vi "Draw 2D Plot.vi"(6 "Control Ref Queue":T1, 8 "error in (no error)":errorcluster, 10 "Multiplot Representation In":T2, 11 "2D Error Bar.lvclass in":refnum<class "2D Error Bar.lvclass">) -> (0 "error out":errorcluster, 2 "Multiplot Representation Out":T2, 3 "2D Error Bar.lvclass out":refnum<class "2D Error Bar.lvclass">)   [LabVIEW 2020, in "2D Error Bar.lvclass"]
uses:
  <vilib>/Math Plots/2D Math Plots/2D Error Bar/2D Error Bar/2D Error Bar.lvclass
  e:/builds/penguin/labview/branches/2020/dev/dist/vi.lib/Math Plots/2D Math Plots/2D Plot/2D Plot/2D Plot.lvclass
  <vilib>/Math Plots/2D Math Plots/2D Plot/2D Plot/Typedef/Multiplot Representation.ctl
  <vilib>/Math Plots/2D Math Plots/2D Plot/2D Plot/Typedef/Plot Representation.ctl
  <vilib>/Math Plots/2D Math Plots/2D Plot/2D Plot/Typedef/Range Cluster.ctl
  <vilib>/Math Plots/2D Math Plots/2D Plot/Action String/2DMathPlot Ctrl Act Queue.ctl
  <vilib>/Math Plots/2D Math Plots/2D Plot/Action String/2DMathPlot Ctrl Act Cluster.ctl
  <vilib>/Math Plots/2D Math Plots/2D Plot/Action String/2DMathPlot State Class.ctl
  <vilib>/Math Plots/2D Math Plots/2D Error Bar/2D Error Bar/2D Error Bar.lvclass/2D Error Bar.ctl
  <vilib>/Math Plots/2D Math Plots/2D Plot/2D Plot/2D Plot.lvclass
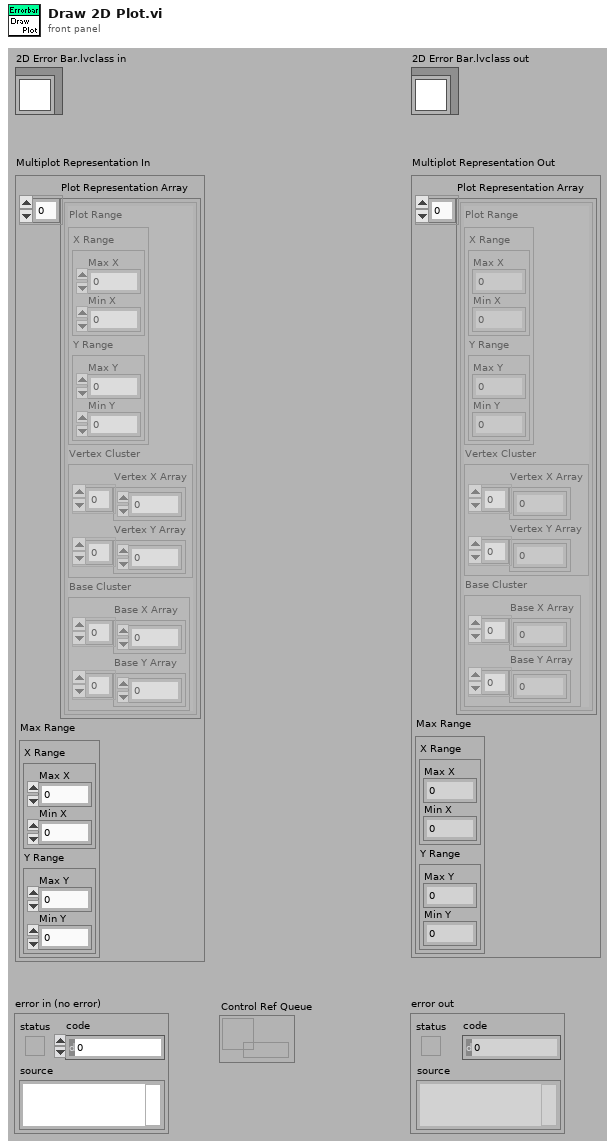
[diagram p1: front panel]
types:
  T1 = typedef "2DMathPlot Ctrl Act Queue.ctl" = refnum<queue>
  T2 = typedef "2D Plot.lvclass/Multiplot Representation.ctl" = cluster{"Plot Representation Array":T3[], "Max Range":T4}
  T3 = typedef "2D Plot.lvclass/Plot Representation.ctl" = cluster{"Plot Range":T4, "Vertex Cluster":cluster{"Vertex X Array":dbl[], "Vertex Y Array":dbl[]}, "Base Cluster":cluster{"Base X Array":dbl[], "Base Y Array":dbl[]}}
  T4 = typedef "2D Plot.lvclass/Range Cluster.ctl" = cluster{"X Range":cluster{"Max X":dbl, "Min X":dbl}, "Y Range":cluster{"Max Y":dbl, "Min Y":dbl}}
  T5 = typedef "2DMathPlot Ctrl Act Cluster.ctl" = cluster{"Plot Area Ref":refnum<vi>, "Z Axis Ref":refnum<vi>, "Legend Ref":refnum<vi>, "XControl Ref":refnum<vi>, "Facade Ref":refnum<vi>, "Display State Change Class":T6}
  T6 = typedef "2DMathPlot State Class.ctl" = enum16{"Update All (Undo)", "Update General", "Update Appearance", "Update Format", "Update Scale", "Update Marker", "Update Cursor", "None"}
  T7 = cluster{"Base X Array":dbl[], "Base Y Array":dbl[]}
  T8 = typedef "2D Plot.lvclass/Plot Property Array.ctl" = T9[]
  T9 = typedef "2D Plot.lvclass/Plot Property.ctl" = cluster{"Bar Plot Style":u8, "DigitalLineStyle":u8, "TransitionLocation":u8, "Transition Type":u8, "Fill To":i16, "Fill/Pt. Color":u32, "Label Style":u8, "Line Style":u8, "Line Width":u8, "Plot Color":u32, "Plot Interpolation":u8, "Plot Name":string, "Point Style":u8, "Visible?":bool, "XScaleIdx":u32, "YScaleIdx":u32}
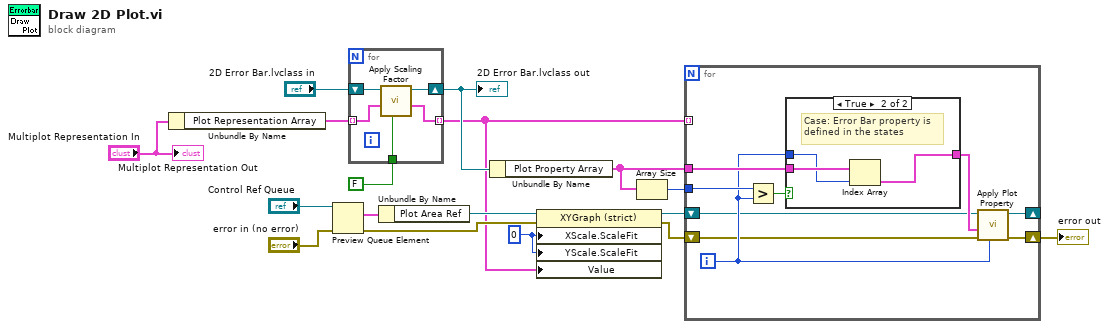
[diagram p0: block diagram]
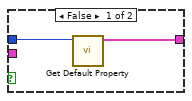
[diagram p2: hidden frame]
diagram:
  w11 = u8 0 ("X Scale.Scale Fit")
  n1 = Unbundle By Name("Multiplot Representation In") -> ("Plot Representation Array"=w5:T3[])
  n2 = Preview Queue Element(queue="Control Ref Queue", error in (no error)="error in (no error)") -> (element=w8:T5, error out=w10:errorcluster)  [unwired: 3 out]
  n3 = for {
    tunnel: w5 -> [w22] mode=indexing
    tunnel: [w18] -> w1 mode=indexing
    tunnel: FALSE ("Plot Image?") -> [w21]
    shift-right: [w19] -> w2
    shift-left: "2D Error Bar.lvclass in" -> [w20]
    n4 = call <vilib>:"Apply Scaling Factor.vi"("Apply to Vertex?"=w21, "Plot Representation Cluster"=w22, "2D Plot.lvclass in"=w20) -> ("Base Cluster"=w18:T7, "2D Plot.lvclass out"=w19:refnum<class "2D Error Bar.lvclass">)  [unwired: 1 in, 6 out]
  }
  "2D Error Bar.lvclass out" <- w2
  n5 = Unbundle By Name(w8) -> ("Plot Area Ref"=w16:refnum<vi>)
  n6 = Unbundle By Name(w2) -> ("Plot Property Array"=w15:T8)
  n7 = property class="XYGraph (strict)"(reference=w16, error in=w10, "XScale.ScaleFit"=w11, "YScale.ScaleFit"=w11, "Value"=w1) -> (reference out=w14:refnum<vi>, error out=w13:errorcluster)
  n8 = Array Size(array=w15) -> (size(s)=w12:i32)
  n9 = for {
    shift-right: [w29] -> _
    shift-left: w14 -> [w23]
    shift-right: [w30] -> w7
    shift-left: w13 -> [w24]
    tunnel: w15 -> [w31]
    tunnel: w12 -> [w28]
    tunnel: w1 -> [_] mode=indexing
    i -> [w26]
    n10 = Greater?(x=w28, y=w26) -> (0:w27:bool)
    n11 = case shown="True" w27 {
      tunnel: w31 -> [_ w36]
      tunnel: w26 -> [w33 w35]
      tunnel: [w32 w34] -> w25
      frame False {
        n12 = call <vilib>:"Get Default Property.vi"("Index"=w33) -> ("Temporary Property"=w32:T9)  [unwired: 4 in, 6 out]
      }
      frame True {
        # "Case: Error Bar property is \ndefined in the states"
        n13 = Index Array(array=w36, index=w35) -> (element=w34:T9)
      }
    }
    n14 = call <vilib>:"Apply Plot Property.vi"("Plot ID"=w26, "error in (no error)"=w24, "Plot Property"=w25, "Polar Area Ref In"=w23) -> ("error out"=w30:errorcluster, "Polar Area Ref Out"=w29:refnum<vi>)  [unwired: 1 in, 5 out]
  }
  "error out" <- w7
  "Multiplot Representation Out" <- "Multiplot Representation In"
